vi "Wait until done.vi"(8 "error in (no error)":errorcluster, 10 "Event Registration":refnum<event-registration>, 11 "Execution API In":refnum<class "Execution API.lvclass">) -> (0 "error out":errorcluster, 2 "Output":string, 3 "Execution API Out":refnum<class "Execution API.lvclass">)   [LabVIEW 2020, in "Execution API.lvclass"]
doc: "Waits until all tests have been executed. The Result Events is obtained from the Register for Events.vi"
uses:
  Execution API.lvclass
  Core/Result/Result.ctl
  Core/Result/Status.ctl
  Core/Result/Type.ctl
  Core/Result/Result.lvlib
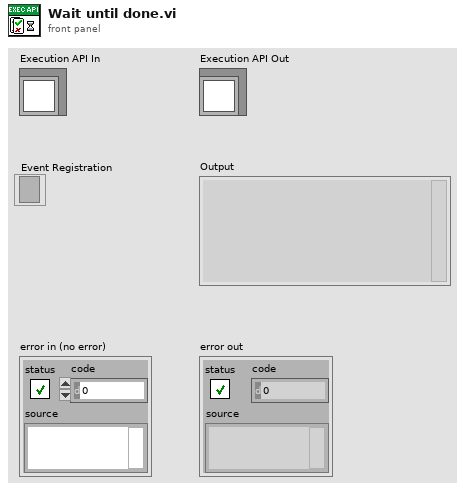
[diagram p1: front panel]
types:
  T1 = typedef "Result.lvlib/Status.ctl" = enum16{"", "Passed", "Failed", "Error", "Skipped", "Setup Error", "Broken", "Teardown Error"}
  T2 = typedef "Result.lvlib/Type.ctl" = enum16{"Test Case", "Test Suite", "Test Run", "Pass", "Fail", "Skip", "Pass if", "Fail if", "Pass if Error", "Fail if Error", "Pass if Equal", "Fail if Equal"}
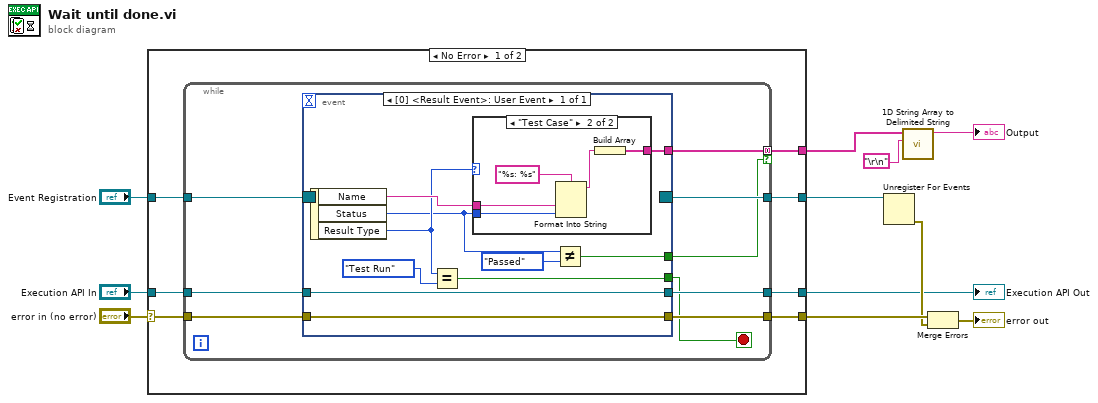
[diagram p0: block diagram]
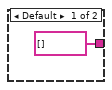
[diagram p2: hidden frame]
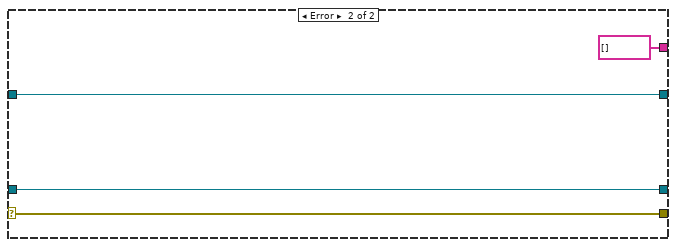
[diagram p3: hidden frame]
diagram:
  n1 = case shown="No Error" "error in (no error)" {
    selector: "error in (no error)" -> [w16 w47]
    tunnel: [w12 string[] []] -> w11
    tunnel: "Execution API In" -> [w18 w46]
    tunnel: [w17 w46] -> w1
    tunnel: [w15 w47] -> w7
    tunnel: [w14 w45] -> w2
    tunnel: "Event Registration" -> [w13 w45]
    frame No Error {
      n2 = while {
        tunnel: w13 -> [w27]
        tunnel: w16 -> [w24]
        tunnel: w18 -> [w25]
        tunnel: [w23] -> w17
        tunnel: [w22] -> w15
        tunnel: [w26] -> w14
        tunnel: [w20] -> w12 mode=concatenating if=w19
        stop <- w21 stop-if-true
        n3 = event shown="[0] <Result Event>: User Event" {
          selector: w27 -> [_]
          dyn-events: [_] -> w26
          timeout: _ -> [_]
          tunnel: w25 -> [w28]
          tunnel: w24 -> [w37]
          tunnel: [w28] -> w23
          tunnel: [w37] -> w22
          tunnel: [w35] -> w21
          tunnel: [w33] -> w20
          tunnel: [w29] -> w19
          event User Event {
            n4 = event-data() -> ("Name"=w34:string, "Status"=w31:T1, "Result Type"=w32:T2)  [unwired: 1 in]
            n5 = Equal?(x=w32, y=Type."Test Run") -> (x = y?=w35:bool)
            n6 = case shown="\"Test Case\"" w32 {
              tunnel: w34 -> [_ w42]
              tunnel: w31 -> [_ w41]
              tunnel: [string[] [] w39] -> w33
              frame Default {
              }
              frame "Test Case" {
                n7 = Format Into String(format string="%s: %s", w42, w41) -> (resulting string=w40:string)  [unwired: 2 in, 1 out]
                n8 = Build Array(w40) -> (w39:string[])
              }
            }
            n9 = Not Equal?(x=w31, y=Status."Passed") -> (x != y?=w29:bool)
          }
        }
      }
    }
    frame Error {
    }
  }
  "Execution API Out" <- w1
  n10 = Unregister For Events(event registration refnum=w2) -> (error out=w4:errorcluster)  [unwired: 1 in]
  n11 = call <vilib>:"1D String Array to Delimited String.vi"("delimiter"="\r\n", "string array"=w11) -> ("delimited string"=→"Output":string)  [unwired: 9 in]
  n12 = Merge Errors(w7, w4) -> (→"error out":errorcluster)
